vi "FGV Temp.vi"(5 "Temp_Unit":T1, 9 "action":enum16{"set", "get"}(ring)) -> (6 "Temp_Unit 2":T1)   [LabVIEW 2014, in "FH 55.lvlib"]
doc: "In dieser FGV wird die ausgewählte Temperaturausgabe gespeichert:\n keine Temperaturausgabe \n Temperaturausgabe in Celsius\n Temperaturausgabe in Fahrenheit\n\n\nIn this FGV the selected temperature output is saved:\n No temperature output\n Output temperature in Celsius\n Output temperature in Fahrenheit"
uses:
  FH 55.lvlib
  TypeDef/Temp_Unit.ctl
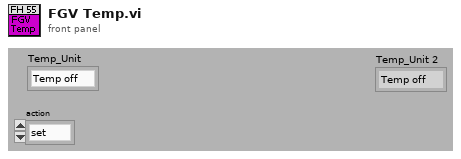
[diagram p1: front panel]
types:
  T1 = typedef "FH 55.lvlib/Temp_Unit.ctl" = enum16{"Temp off", "Celsius", "Fahrenheit"}
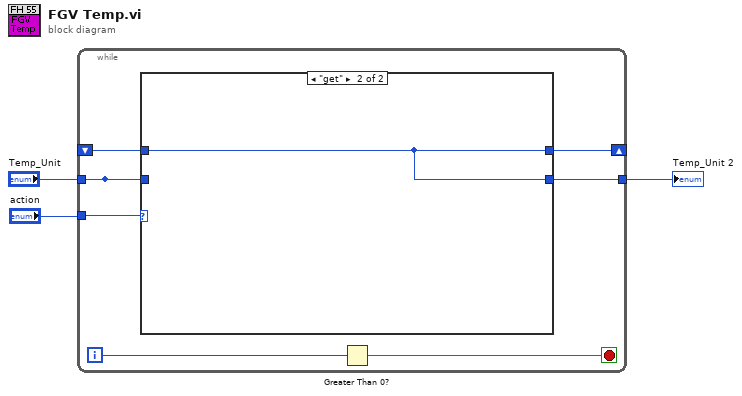
[diagram p0: block diagram]
diagram:
  n1 = while {
    tunnel: "Temp_Unit" -> [w9]
    tunnel: [w9] -> _
    shift-right: [w7] -> _
    shift-left: _ -> [w10]
    tunnel: [w8] -> w1
    tunnel: "action" -> [w4]
    i -> [w6]
    stop <- w5 stop-if-true
    n2 = case shown="\"get\"" w4 {
      tunnel: w10 -> [_ w12]
      tunnel: w9 -> [w11 _]
      tunnel: [w11 w12] -> w8
      tunnel: [w11 w12] -> w7
      frame "set", Default {
      }
      frame "get" {
      }
    }
    n3 = Greater Than 0?(x=w6) -> (x > 0?=w5:bool)
  }
  "Temp_Unit 2" <- w1
